vi "Write_Spread_Flo.vi"() -> ()   [LabVIEW 2014]
uses:
  <vilib>/Utility/file.llb/Write To Spreadsheet File (I64).vi
  <vilib>/Utility/file.llb/Read From Spreadsheet File (DBL).vi
panel:
  out "Show Range":enum8{"10", "20", "40", "80"}[](array[ring])=[enum."80", enum."80", enum."80", enum."80", enum."80", enum."80", enum."80", enum."80", enum."80", enum."80", enum."80", enum."80", enum."80", enum."80", enum."80", enum."80", enum."80", enum."80", enum."80", enum."80", enum."80", enum."80", enum."80", enum."80", enum."80", enum."80", enum."80", enum."80", enum."80", enum."80", enum."80", enum."80", enum."80", enum."80", enum."80", enum."80", enum."80", enum."80", enum."80", enum."80", enum."80", enum."80", enum."80", enum."80", enum."80", enum."80", enum."80", enum."80", enum."80", enum."80", enum."80", enum."80", enum."80", enum."80", enum."80", enum."80", enum."80", enum."80", enum."80", enum."80", enum."80", enum."80", enum."80", enum."80", enum."80", enum."80", enum."80", enum."80", enum."80", enum."80", enum."80", enum."80", enum."80", enum."80", enum."80", enum."80", enum."80", enum."80", enum."80", enum."80", enum."80", enum."80", enum."80", enum."80", enum."80", enum."80", enum."80", enum."80", enum."80", enum."80", enum."80", enum."80", enum."80", enum."80", enum."80", enum."80", enum."80", enum."80", enum."80", enum."80", enum."80", enum."80", enum."80", enum."80", enum."80", enum."80", enum."80", enum."80", enum."80", enum."80", enum."80", enum."80", enum."80", enum."80", enum."80", enum."80", enum."80", enum."80", enum."80", enum."80", enum."80", enum."80", enum."80", enum."80", enum."80", enum."80", enum."80", enum."80"]
  in  "file path (dialog if empty)":path=path "C:/W7-X-DAQ-Data/_DAQ_Ranges.txt"
  in  "Write Range":enum8{"10", "20", "40", "80"}[](array[ring])=[enum."80", enum."80", enum."80", enum."80", enum."80", enum."80", enum."80", enum."80", enum."80", enum."80", enum."80", enum."80", enum."80", enum."80", enum."80", enum."80", enum."80", enum."80", enum."80", enum."80", enum."80", enum."80", enum."80", enum."80", enum."80", enum."80", enum."80", enum."80", enum."80", enum."80", enum."80", enum."80", enum."80", enum."80", enum."80", enum."80", enum."80", enum."80", enum."80", enum."80", enum."80", enum."80", enum."80", enum."80", enum."80", enum."80", enum."80", enum."80", enum."80", enum."80", enum."80", enum."80", enum."80", enum."80", enum."80", enum."80", enum."80", enum."80", enum."80", enum."80", enum."80", enum."80", enum."80", enum."80", enum."80", enum."80", enum."80", enum."80", enum."80", enum."80", enum."80", enum."80", enum."80", enum."80", enum."80", enum."80", enum."80", enum."80", enum."80", enum."80", enum."80", enum."80", enum."80", enum."80", enum."80", enum."80", enum."80", enum."80", enum."80", enum."80", enum."80", enum."80", enum."80", enum."80", enum."80", enum."80", enum."80", enum."80", enum."80", enum."80", enum."80", enum."80", enum."80", enum."80", enum."80", enum."80", enum."80", enum."80", enum."80", enum."80", enum."80", enum."80", enum."80", enum."80", enum."80", enum."80", enum."80", enum."80", enum."80", enum."80", enum."80", enum."80", enum."80", enum."80", enum."80", enum."80", enum."80", enum."80"]
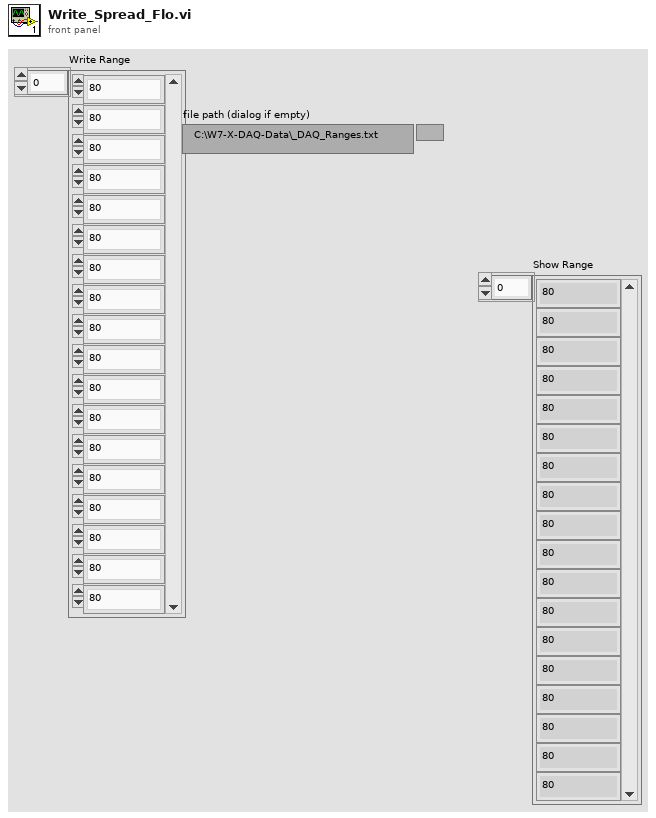
[diagram p1: front panel]
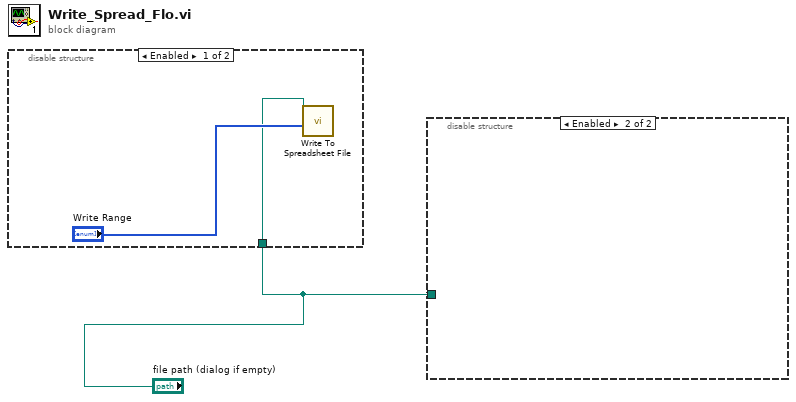
[diagram p0: block diagram]
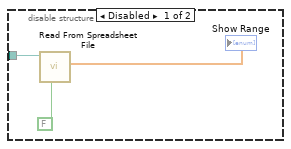
[diagram p2: hidden frame]
diagram:
  n1 = disable-structure shown="Enabled" {
    disable-tunnel: "file path (dialog if empty)" -> [w2 _]
    frame Enabled {
      n2 = call-poly <vilib>:"Write To Spreadsheet File.vi"("1D data"="Write Range", "file path (dialog if empty)"=w2) -> ()  [unwired: 6 in, 1 out]
    }
    frame Disabled {
    }
  }
  n3 = disable-structure shown="Enabled" {
    disable-tunnel: "file path (dialog if empty)" -> [w6 _]
    frame Disabled {
      n4 = call-poly <vilib>:"Read From Spreadsheet File.vi"("transpose (no:F)"=FALSE, "file path (dialog if empty)"=w6) -> ("first row"=→"Show Range":dbl[])  [unwired: 5 in, 4 out]
    }
    frame Enabled {
    }
  }
